vi "GetTableColumns.vi"() -> ()   [LabVIEW 2018]
uses:
  <vilib>/addons/database/Auxilliary.llb/DB Tools DataTypes.ctl
  <vilib>/addons/database/Connection.llb/DB Tools Open Connec (Path).vi
  <vilib>/addons/database/NI_Database_API.lvlib
panel:
  out "columns":string[](array[string])=["ID", "cMacCode", "cInvCode", "cCheckDate", "cCheckNo", "cState", "cDefine1", "cDefine2", "cDefine3", "cDefine4", "cDefine5", "cDefine6", "cDefine7", "cDefine8", "cDefine9", "cDefine10", "cDefine11", "cDefine12", "cDefine13", "cDefine14", "cDefine15", "cDefine16", "cDefine17", "cDefine18", "CreateDate"]
  out "column information":T2(array[cluster])=[{"name"="ID", "database data type"=enum."Long (I32)", "defined size"=4}, {"name"="cMacCode", "database data type"=enum."String", "defined size"=20}, {"name"="cInvCode", "database data type"=enum."String", "defined size"=40}, {"name"="cCheckDate", "database data type"=enum."Date/Time", "defined size"=16}, {"name"="cCheckNo", "database data type"=enum."String", "defined size"=40}, {"name"="cState", "database data type"=enum."String", "defined size"=10}, {"name"="cDefine1", "database data type"=enum."String", "defined size"=10}, {"name"="cDefine2", "database data type"=enum."String", "defined size"=10}, {"name"="cDefine3", "database data type"=enum."String", "defined size"=10}, {"name"="cDefine4", "database data type"=enum."String", "defined size"=10}, {"name"="cDefine5", "database data type"=enum."String", "defined size"=10}, {"name"="cDefine6", "database data type"=enum."String", "defined size"=10}, {"name"="cDefine7", "database data type"=enum."Double (DBL)", "defined size"=19}, {"name"="cDefine8", "database data type"=enum."String", "defined size"=10}, {"name"="cDefine9", "database data type"=enum."Double (DBL)", "defined size"=19}, {"name"="cDefine10", "database data type"=enum."Double (DBL)", "defined size"=19}, {"name"="cDefine11", "database data type"=enum."Double (DBL)", "defined size"=19}, {"name"="cDefine12", "database data type"=enum."Double (DBL)", "defined size"=19}, {"name"="cDefine13", "database data type"=enum."Double (DBL)", "defined size"=19}, {"name"="cDefine14", "database data type"=enum."Double (DBL)", "defined size"=19}, {"name"="cDefine15", "database data type"=enum."String", "defined size"=50}, {"name"="cDefine16", "database data type"=enum."String", "defined size"=50}, {"name"="cDefine17", "database data type"=enum."String", "defined size"=50}, {"name"="cDefine18", "database data type"=enum."String", "defined size"=50}, {"name"="CreateDate", "database data type"=enum."Date/Time", "defined size"=16}]
  out "error out":errorcluster
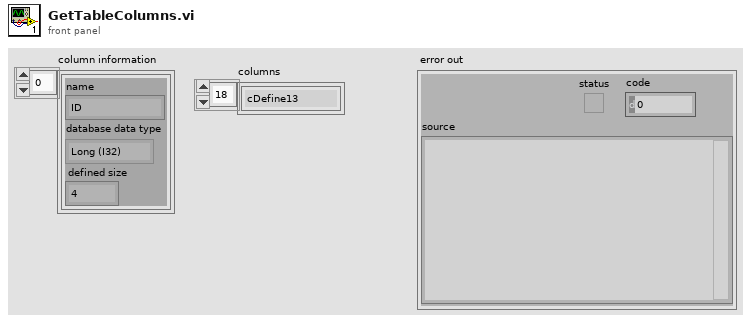
[diagram p1: front panel]
types:
  T1 = typedef "NI_Database_API.lvlib/DB Tools DataTypes.ctl" = enum16{"String", "Long (I32)", "Single (SGL)", "Double (DBL)", "Date/Time", "Binary"}
  T2 = cluster{"name":string, "database data type":T1, "defined size":i32}[]
  T3 = typedef "NI_Database_API.lvlib/Conn ObjectReference.ctl" = refnum<k1>
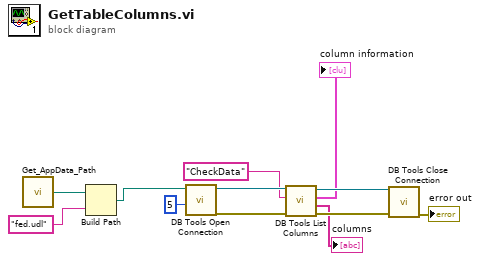
[diagram p0: block diagram]
diagram:
  n1 = call "Get_AppData_Path.vi"() -> ("path"=w11:path)  [unwired: 1 in]
  n2 = Build Path(base path=w11, name or relative path="fed.udl" ("名称或相对路径")) -> (appended path=w10:path)
  n3 = call-poly <vilib>:"DB Tools Open Connection.vi"("connection timeout (15)"=5, "connection information"=w10) -> ("error out"=w5:errorcluster, "connection reference"=w7:T3)  [unwired: 6 in]
  n4 = call <vilib>:"DB Tools List Columns.vi"("error in (no error)"=w5, "table"="CheckData", "connection reference"=w7) -> ("error out"=w4:errorcluster, "columns"=→"columns":string[], "column information"=→"column information":T2, "connection reference out"=w6:T3)  [unwired: 1 in]
  n5 = call <vilib>:"DB Tools Close Connection.vi"("error in (no error)"=w4, "connection reference"=w6) -> ("error out"=→"error out":errorcluster)  [unwired: 5 in]
